vi "GUILib.simple boolean init.vi"(0 "ctlRef":refnum<vi>, 5 "error in (no error)":errorcluster) -> (14 "ctlRef dup":refnum<vi>, 19 "error out":errorcluster)   [LabVIEW 2012, in "GUILib.lvlib"]
doc: "initialiazes a specific type of control by setting default values"
uses:
  GUILib.lvlib
  UtilityLib/UtilityLib.valueStatus.ctl
  UtilityLib/UtilityLib.lvlib
panel:
  in  "booleanType":bool
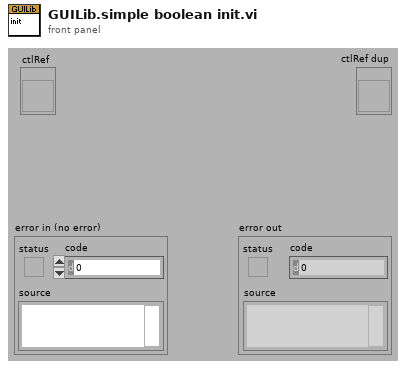
[diagram p1: front panel]
types:
  T1 = typedef "UtilityLib.lvlib/UtilityLib.valueStatus.ctl" = enum16{"no info available", "stand by/off", "on", "warning", "alarm/malfunction", "not implemented", "user action required", "important information", "system default", "control default", "indicator default", "button default"}
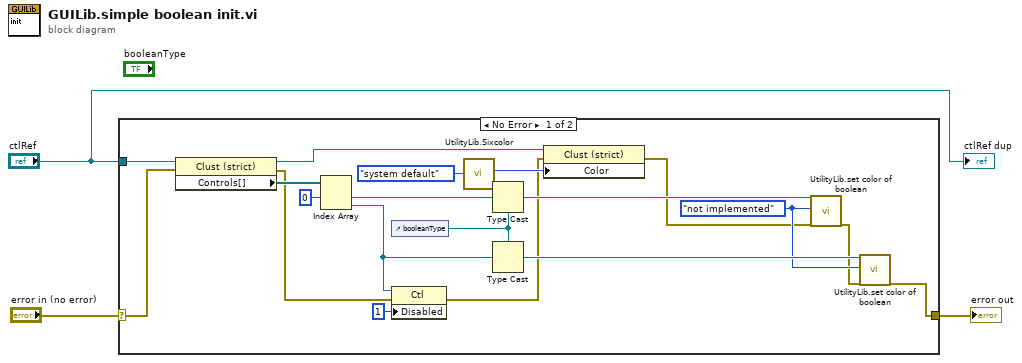
[diagram p0: block diagram]
diagram:
  n1 = case shown="No Error" "error in (no error)" {
    selector: "error in (no error)" -> [w17 w23]
    tunnel: "ctlRef" -> [w18 _]
    tunnel: [w4 w23] -> w2
    frame No Error {
      w8 = UtilityLib.valueStatus."not implemented" ("valueStatus")
      n2 = property on="Property Node" class="Clust (strict)"(reference=w18, error in=w17) -> (reference out=w15:refnum<vi>, error out=w16:errorcluster, "Controls[]"=w19:refnum<vi>[])
      n3 = Index Array(array=w19, index #1=0 ("index")) -> (element #1=w22:refnum<vi>, element #2=w10:refnum<vi>)  [unwired: 1 in]
      n4 = control-ref of="booleanType"() -> (w11:refnum<vi>)
      n5 = property class="Ctl"(reference=w10, error in=w16, "Disabled"=u8 1) -> (error out=w7:errorcluster)  [unwired: 1 out]
      n6 = call "UtilityLib.Sixcolor.vi"("State"=UtilityLib.valueStatus."system default") -> ("elementBackground"=w14:u32)  [unwired: 2 in, 3 out]
      n7 = Type Cast(type=w11, x=w22) -> (*(type *) &x=w12:refnum<vi>)
      n8 = Type Cast(type=w11, x=w10) -> (*(type *) &x=w9:refnum<vi>)
      n9 = property on="Property Node" class="Clust (strict)"(reference=w15, error in=w7, "Color"=w14) -> (error out=w6:errorcluster)  [unwired: 1 out]
      n10 = call "UtilityLib.set color of boolean.vi"("button"=w12, "valueStatus"=w8, "error in (no error)"=w6) -> ("error out"=w5:errorcluster)  [unwired: 16 in]
      n11 = call "UtilityLib.set color of boolean.vi"("button"=w9, "valueStatus"=w8, "error in (no error)"=w5) -> ("error out"=w4:errorcluster)  [unwired: 16 in]
    }
    frame Error {
    }
  }
  "error out" <- w2
  "ctlRef dup" <- "ctlRef"
